vi "construct.vi"(8 "error in (no error)":errorcluster, 9 "configuration name":string, 10 "load config file? (T)":bool=TRUE, 11 "GenericPlugin in":refnum<class "TrajectoryMH100122AODRAPS.lvclass">) -> (0 "error out":errorcluster, 3 "GenericPlugin out":refnum<class "TrajectoryMH100122AODRAPS.lvclass">)   [LabVIEW 2010, in "TrajectoryMH100122AODRAPS.lvclass"]
uses:
  TrajectoryMH100122AODRAPS.lvclass
  TrajectoryMG100122GenericFPGA/TrajectoryMG100122GenericFPGA/TrajectoryMG100122GenericFPGA.lvclass
  FPGAWrapper/GenericFPGAWrapper/GenericFPGAWrapper/GenericFPGAWrapper.lvclass
  TrajectoryMH100122AODRAPS.lvclass/TrajectoryMH100122AODRAPS.ctl
  common/classes/ErrorController/ErrorController/class_data.vi
  common/classes/ErrorController/ErrorController/ErrorController.lvclass
  common/classes/GenericComponent/GenericComponent/GenericComponent.lvclass
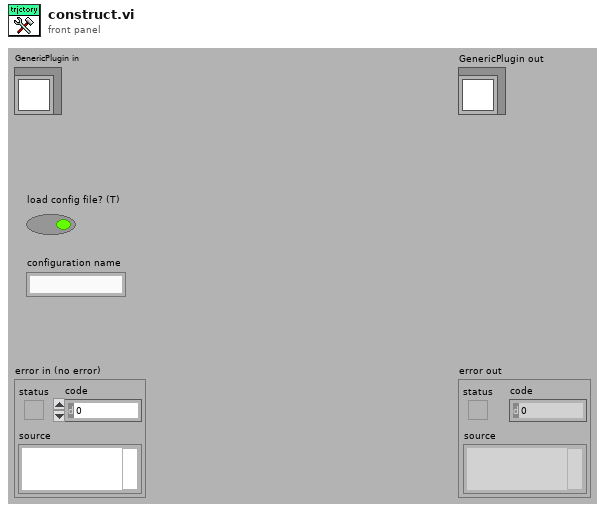
[diagram p1: front panel]
types:
  T1 = cluster{"class path":string, "configuration":string, "label":string, "settings name":string}
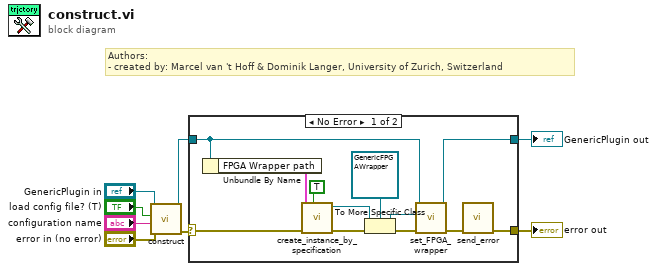
[diagram p0: block diagram]
diagram:
  # "Authors: \n- created by: Marcel van 't Hoff & Dominik Langer, University of Zurich, Switzerland"
  n1 = call-parent "construct.vi"("error in (no error)"="error in (no error)", "configuration name"="configuration name", "load config file?"="load config file? (T)", "GenericPlugin in"="GenericPlugin in") -> ("error out"=w4:errorcluster, "GenericPlugin out"=w3:refnum<class "TrajectoryMH100122AODRAPS.lvclass">)  [unwired: 6 in]
  n2 = case shown="No Error" w4 {
    selector: w4 -> [w13 w21]
    tunnel: w3 -> [w18 w22]
    tunnel: [w14 w21] -> w2
    tunnel: [w16 w22] -> w1
    frame No Error {
      n3 = Unbundle By Name(w18) -> ("FPGA Wrapper path"=w11:T1)
      n4 = call "create_instance_by_specification.vi"("call constructor?"=TRUE, "error in (no error)"=w13, "component specification"=w11) -> ("error out"=w12:errorcluster, "GenericPlugin out"=w10:refnum<class "GenericComponent.lvclass">)  [unwired: 6 in, 1 out]
      n5 = To More Specific Class(target class=refnum<class "GenericFPGAWrapper.lvclass"> refnum ("GenericFPGAWrapper.lvclass"), reference=w10, error in=w12) -> (specific class reference=w19:refnum<class "GenericFPGAWrapper.lvclass">, error out=w17:errorcluster)
      n6 = call-dynamic "set_FPGA_wrapper.vi"("error in (no error)"=w17, "GenericFPGAWrapper.lvclass"=w19, "TrajectoryMG100122GenericFPGA in"=w18) -> ("error out"=w15:errorcluster, "TrajectoryMG100122GenericFPGA out"=w16:refnum<class "TrajectoryMH100122AODRAPS.lvclass">)  [unwired: 7 in]
      n7 = call "send_error.vi"("error in (no error)"=w15) -> ("error out"=w14:errorcluster)  [unwired: 10 in]
    }
    frame Error {
    }
  }
  "error out" <- w2
  "GenericPlugin out" <- w1
